vi "setLaserChannelVisible.vi"(0 "CmbBox Refnum":refnum<vi>, 1 "CmbBox Refnum 2":refnum<vi>, 2 "CmbBox Refnum 3":refnum<vi>, 3 "CmbBox Refnum 4":refnum<vi>, 4 "CmbBox Refnum 5":refnum<vi>, 5 "CmbBox Refnum 6":refnum<vi>, 6 "DigNum Refnum 8":refnum<vi>, 7 "CmbBox Refnum 7":refnum<vi>, 8 "error out 2":errorcluster, 9 "CmbBox Refnum 8":refnum<vi>, 10 "Wavelength":enum16{"Fixed", "UserDefined"}(ring), 11 "DigNum Refnum":refnum<vi>, 13 "DigNum Refnum 2":refnum<vi>, 15 "DigNum Refnum 7":refnum<vi>, 16 "DigNum Refnum 6":refnum<vi>, 17 "DigNum Refnum 5":refnum<vi>, 18 "DigNum Refnum 4":refnum<vi>, 19 "DigNum Refnum 3":refnum<vi>) -> (14 "error out":errorcluster)   [LabVIEW 2011]
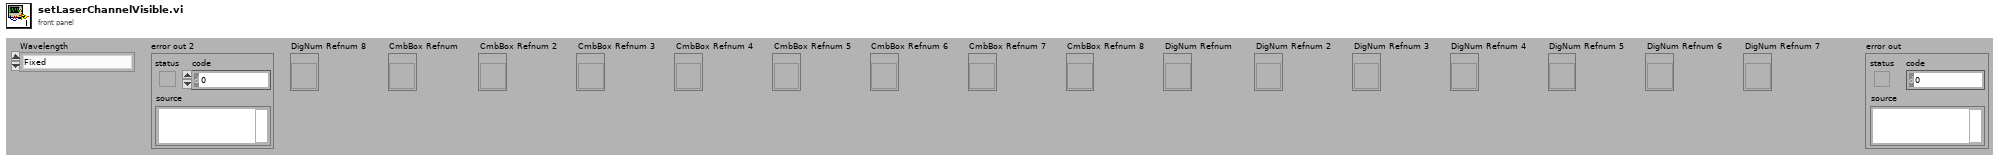
[diagram p1: front panel]
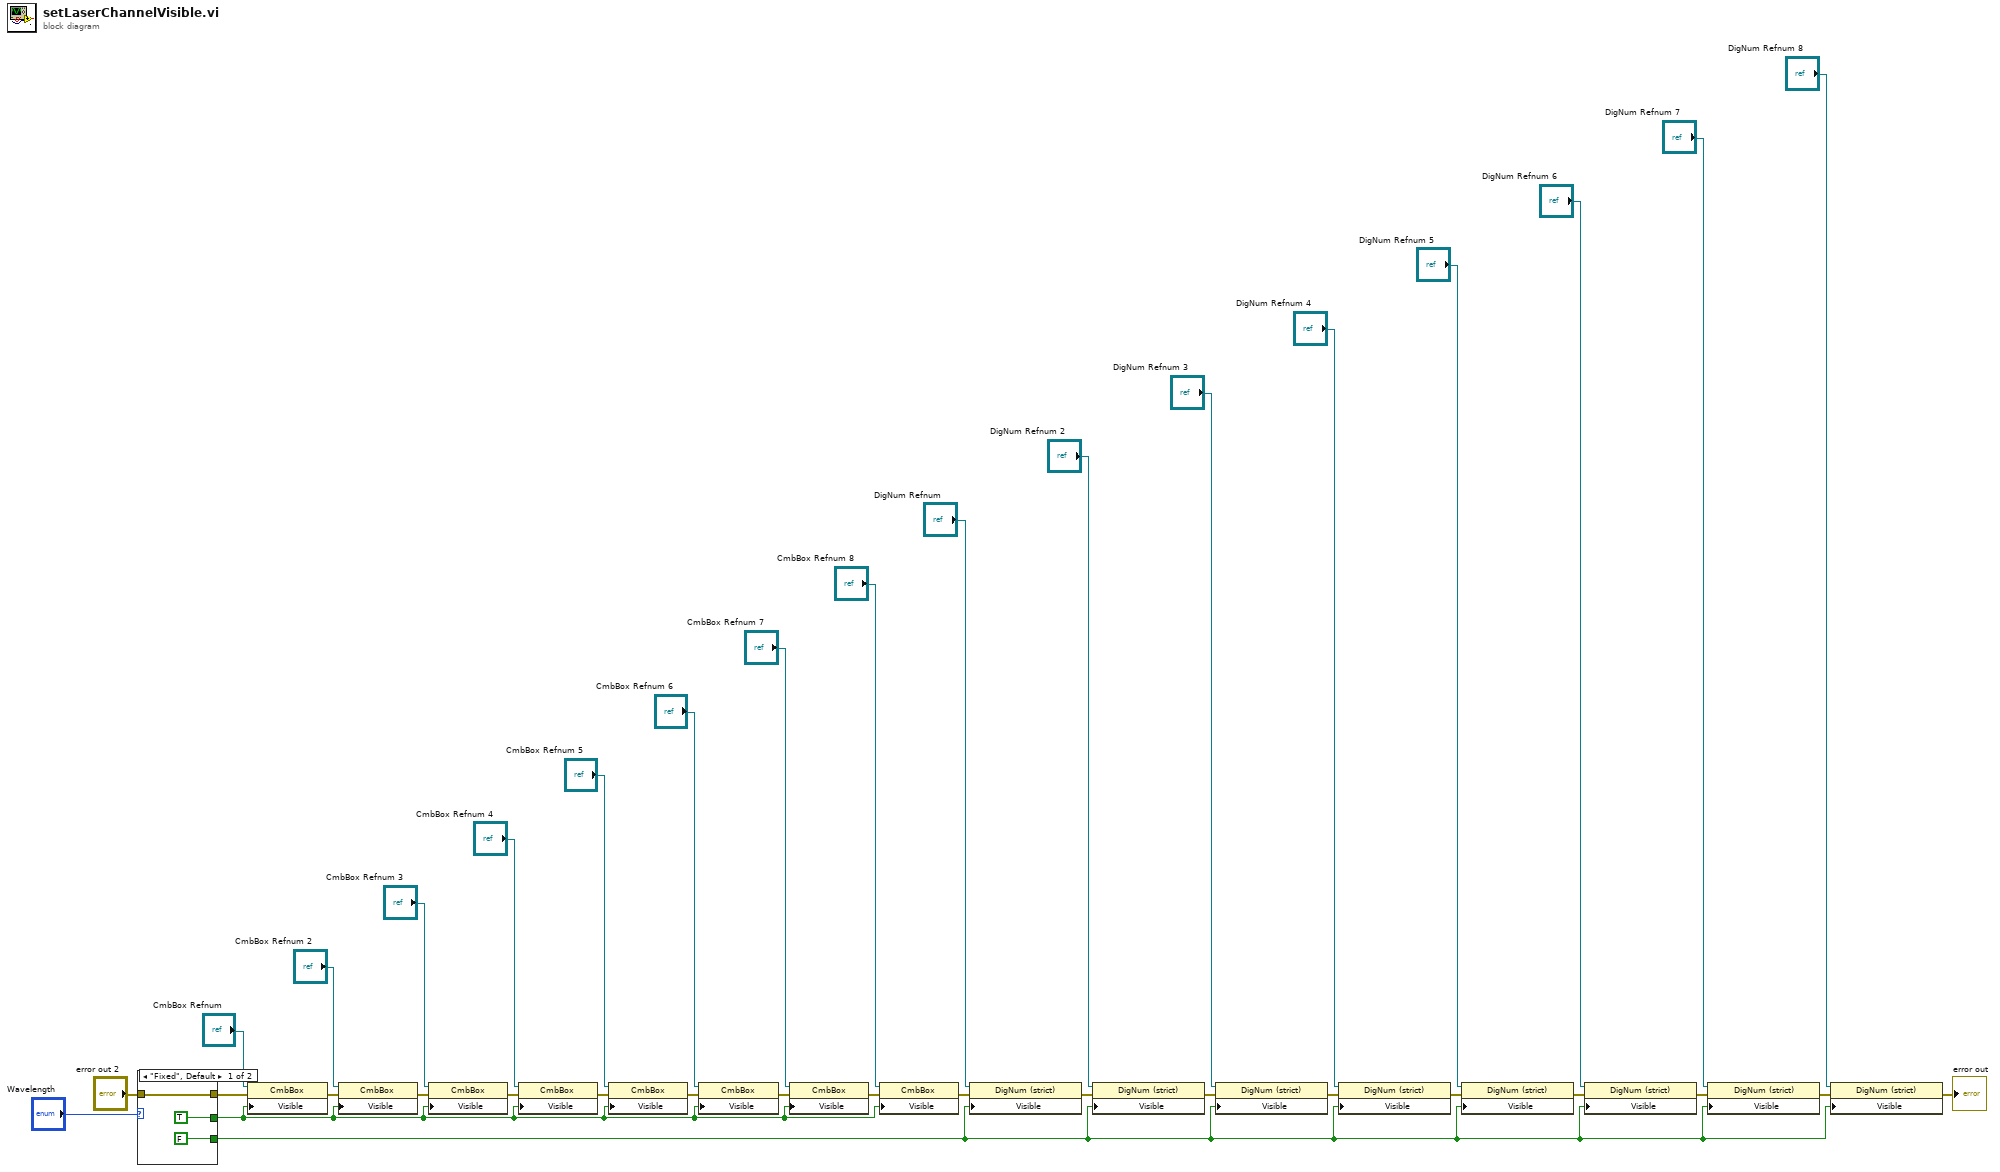
[diagram p0: block diagram]
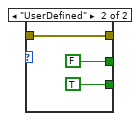
[diagram p2: hidden frame]
diagram:
  n1 = case shown="\"Fixed\", Default" "Wavelength" {
    tunnel: "error out 2" -> [w38 w41]
    tunnel: [TRUE ("Visible") FALSE ("Visible")] -> w34
    tunnel: [FALSE ("Visible") TRUE ("Visible")] -> w35
    tunnel: [w38 w41] -> w37
    frame "Fixed", Default {
    }
    frame "UserDefined" {
    }
  }
  n2 = property on="Property Node" class="CmbBox"(reference="CmbBox Refnum", error in=w37, "Visible"=w34) -> (error out=w19:errorcluster)  [unwired: 1 out]
  n3 = property on="Property Node" class="CmbBox"(reference="CmbBox Refnum 2", error in=w19, "Visible"=w34) -> (error out=w20:errorcluster)  [unwired: 1 out]
  n4 = property on="Property Node" class="CmbBox"(reference="CmbBox Refnum 3", error in=w20, "Visible"=w34) -> (error out=w21:errorcluster)  [unwired: 1 out]
  n5 = property on="Property Node" class="CmbBox"(reference="CmbBox Refnum 4", error in=w21, "Visible"=w34) -> (error out=w22:errorcluster)  [unwired: 1 out]
  n6 = property on="Property Node" class="CmbBox"(reference="CmbBox Refnum 5", error in=w22, "Visible"=w34) -> (error out=w23:errorcluster)  [unwired: 1 out]
  n7 = property on="Property Node" class="CmbBox"(reference="CmbBox Refnum 6", error in=w23, "Visible"=w34) -> (error out=w24:errorcluster)  [unwired: 1 out]
  n8 = property on="Property Node" class="CmbBox"(reference="CmbBox Refnum 7", error in=w24, "Visible"=w34) -> (error out=w25:errorcluster)  [unwired: 1 out]
  n9 = property on="Property Node" class="CmbBox"(reference="CmbBox Refnum 8", error in=w25, "Visible"=w34) -> (error out=w33:errorcluster)  [unwired: 1 out]
  n10 = property on="Property Node" class="DigNum (strict)"(reference="DigNum Refnum", error in=w33, "Visible"=w35) -> (error out=w32:errorcluster)  [unwired: 1 out]
  n11 = property on="Property Node" class="DigNum (strict)"(reference="DigNum Refnum 2", error in=w32, "Visible"=w35) -> (error out=w31:errorcluster)  [unwired: 1 out]
  n12 = property on="Property Node" class="DigNum (strict)"(reference="DigNum Refnum 3", error in=w31, "Visible"=w35) -> (error out=w30:errorcluster)  [unwired: 1 out]
  n13 = property on="Property Node" class="DigNum (strict)"(reference="DigNum Refnum 4", error in=w30, "Visible"=w35) -> (error out=w29:errorcluster)  [unwired: 1 out]
  n14 = property on="Property Node" class="DigNum (strict)"(reference="DigNum Refnum 5", error in=w29, "Visible"=w35) -> (error out=w28:errorcluster)  [unwired: 1 out]
  n15 = property on="Property Node" class="DigNum (strict)"(reference="DigNum Refnum 6", error in=w28, "Visible"=w35) -> (error out=w27:errorcluster)  [unwired: 1 out]
  n16 = property on="Property Node" class="DigNum (strict)"(reference="DigNum Refnum 7", error in=w27, "Visible"=w35) -> (error out=w26:errorcluster)  [unwired: 1 out]
  n17 = property on="Property Node" class="DigNum (strict)"(reference="DigNum Refnum 8", error in=w26, "Visible"=w35) -> (error out=→"error out":errorcluster)  [unwired: 1 out]
